vi "CalibrationDataOrganize.vi"(10 "Calibration Data":dbl[][](array[numeric]), 11 "Data Cluster":T1) -> (1 "min value":dbl, 2 "max value":dbl, 4 "PCAN Calibration DATA":dbl[][](array[numeric]))   [LabVIEW 2026, in "Acquisition.lvlib"]
uses:
  Acquisition.lvlib
  Hardware Configuration.ctl
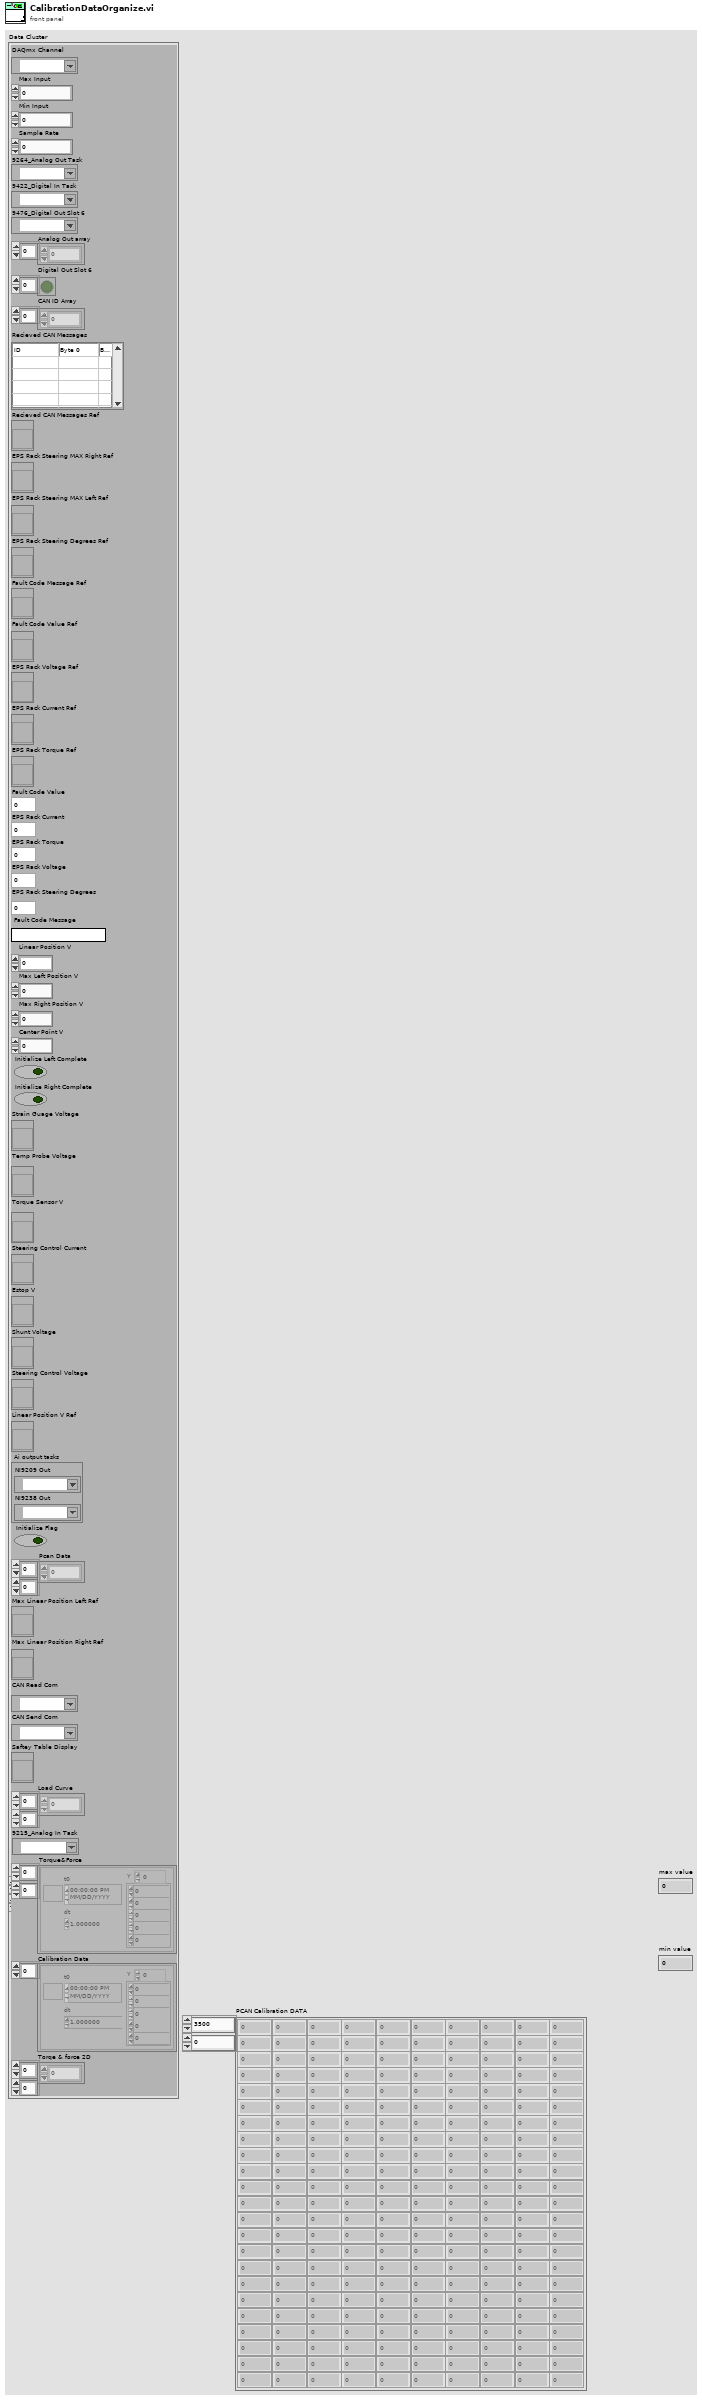
[diagram p1: front panel]
types:
  T1 = typedef "Acquisition.lvlib/Hardware Configuration.ctl" = cluster{"DAQmx Channel":tag, "Max Input":dbl, "Min Input":dbl, "Sample Rate":dbl, "9264_Analog Out Task":refnum<k21>, "9422_Digital In Task":refnum<k21>, "9476_Digital Out Slot 6":refnum<k21>, "Analog Out array":dbl[], "Digital Out Slot 6":bool[], "CAN ID Array":u32[], "Recieved CAN Messages ":string[][], "Recieved CAN Messages Ref":refnum<vi>, "EPS Rack Steering MAX Right Ref":refnum<vi>, "EPS Rack Steering MAX Left Ref":refnum<vi>, "EPS Rack Steering Degrees Ref":refnum<vi>, "Fault Code Message Ref":refnum<vi>, "Fault Code Value Ref":refnum<vi>, "EPS Rack Voltage Ref":refnum<vi>, "EPS Rack Current Ref":refnum<vi>, "EPS Rack Torque Ref":refnum<vi>, "Fault Code Value":dbl, "EPS Rack Current":dbl, "EPS Rack Torque":dbl, "EPS Rack Voltage":dbl, "EPS Rack Steering Degrees":dbl, "Fault Code Message":string, "Linear Position V":dbl, "Max Left Position V":dbl, "Max Right Position V":dbl, "Center Point V":dbl, "Initialize Left Complete":bool, "Initialize Right Complete":bool, "Strain Guage Voltage":refnum<vi>, "Temp Probe Voltage":refnum<vi>, "Torque Sensor V":refnum<vi>, "Steering Control Current":refnum<vi>, "Estop V":refnum<vi>, "Shunt Voltage":refnum<vi>, "Steering Control Voltage":refnum<vi>, "Linear Position V Ref":refnum<vi>, "Ai output tasks":cluster{"NI9209 Out":refnum<k21>, "NI9238 Out":refnum<k21>}, "Initialize Flag":bool, "Pcan Data":dbl[][], "Max Linear Position Left Ref":refnum<vi>, "Max Linear Position Right Ref":refnum<vi>, "CAN Read Com":refnum<k21>, "CAN Send Com":refnum<k21>, "Saftey Table Display":refnum<vi>, "Load Curve":dbl[][], "9215_Analog In Task":refnum<k21>, "Torque&Force":waveform(dbl)[][], "Calibration Data":waveform(dbl)[], "Torqe & force 2D":dbl[][]}
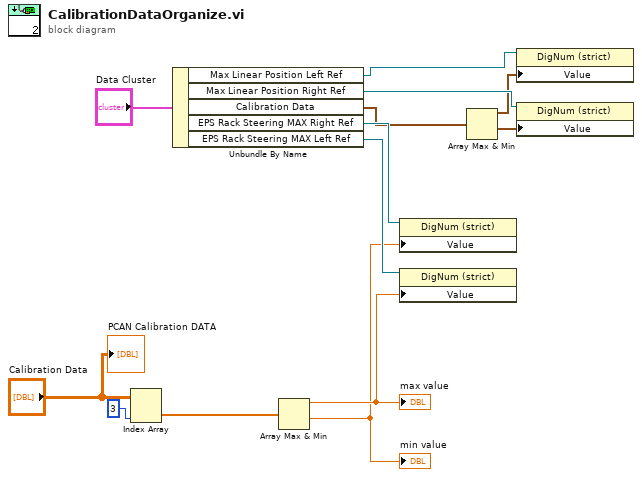
[diagram p0: block diagram]
diagram:
  n1 = Index Array(array="Calibration Data", index (col)=3 ("disabled index (col)")) -> (element=w9:dbl[])  [unwired: 1 in]
  n2 = Unbundle By Name("Data Cluster") -> ("Max Linear Position Left Ref"=w1:refnum<vi>, "Max Linear Position Right Ref"=w5:refnum<vi>, "Calibration Data"=w2:waveform(dbl)[], "EPS Rack Steering MAX Right Ref"=w11:refnum<vi>, "EPS Rack Steering MAX Left Ref"=w12:refnum<vi>)
  n3 = Array Max & Min(array=w9) -> (max value=w13:dbl, min value=w10:dbl)  [unwired: 2 out]
  "max value" <- w13
  "min value" <- w10
  n4 = property class="DigNum (strict)"(reference=w11, "Value"=w10) -> ()  [unwired: 1 in, 2 out]
  n5 = property class="DigNum (strict)"(reference=w12, "Value"=w13) -> ()  [unwired: 1 in, 2 out]
  n6 = Array Max & Min(array=w2) -> (max value=w3:waveform(dbl), min value=w4:waveform(dbl))  [unwired: 2 out]
  n7 = property class="DigNum (strict)"(reference=w1, "Value"=w3) -> ()  [unwired: 1 in, 2 out]
  n8 = property class="DigNum (strict)"(reference=w5, "Value"=w4) -> ()  [unwired: 1 in, 2 out]
  "PCAN Calibration DATA" <- "Calibration Data"
